vi "Start_track.vi"(0 "TCP connection ID":refnum<k5>, 5 "UDP connection ID":refnum<k16>, 7 "IP address in":u32, 11 "Euler Angles DMARS [º] debug":cluster{"phi":dbl, "theta":dbl, "psi":dbl}={"phi"=2.3, "theta"=1.93, "psi"=0.0}, 12 "error in":errorcluster) -> (4 "TCP connection ID out":refnum<k5>, 6 "UDP connection ID out":refnum<k16>, 8 "IP address out":u32, 10 "timeout ms (25000)":i32=1000, 14 "error out":errorcluster)   [LabVIEW 2017]
panel:
  out "outer ini":string
  out "middle ini":string
  out "inner ini":string
  out "String 5":string
  out "String 4":string
  out "String 3":string
  out "String 2":string
  out "String 1":string
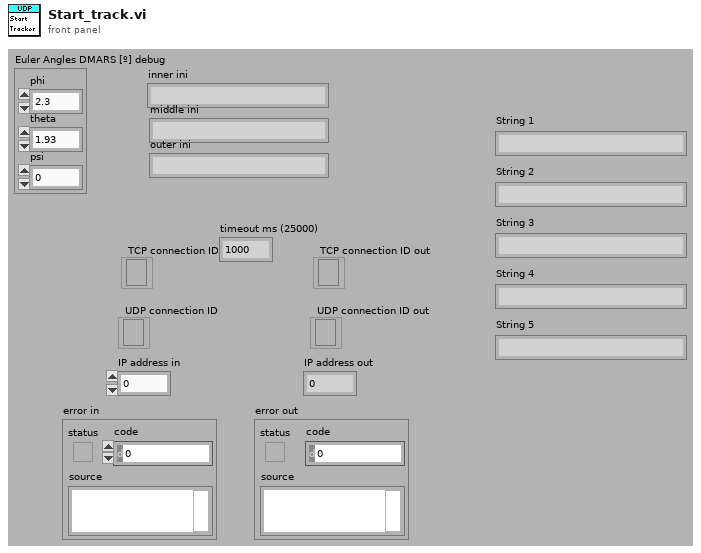
[diagram p1: front panel]
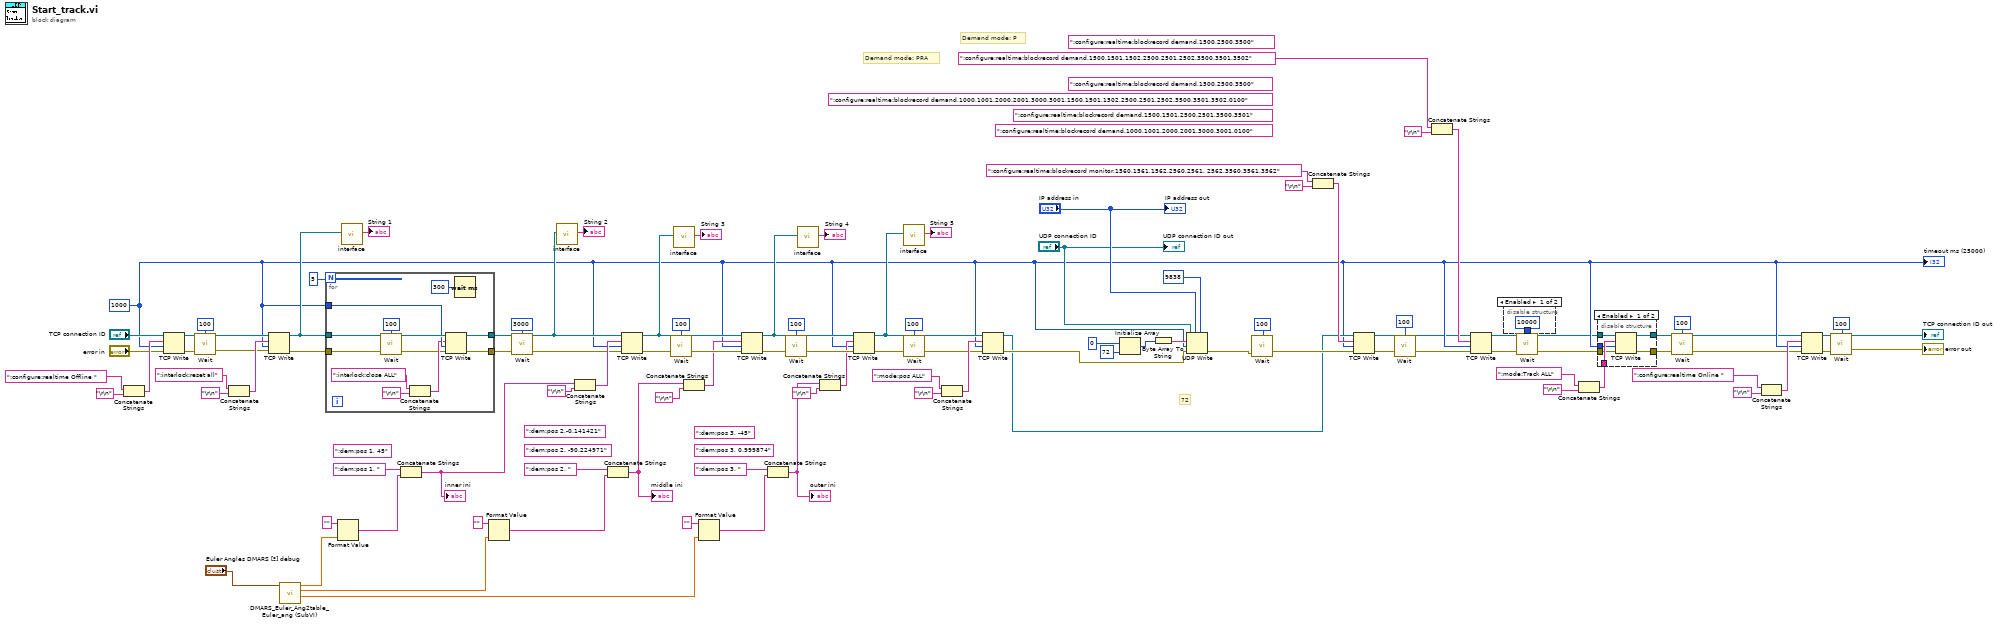
[diagram p0: block diagram]
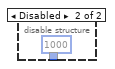
[diagram p3: hidden frame]
diagram:
  (unwired) ":dem:pos 3, 0.999874" ("ACL Command")
  (unwired) ":dem:pos 2, -90.224971" ("ACL Command")
  (unwired) ":dem:pos 3, -45" ("ACL Command")
  (unwired) ":dem:pos 2,-0.141421" ("ACL Command")
  (unwired) ":configure:realtime:blockrecord demand,1500,2500,3500" ("string")
  (unwired) ":configure:realtime:blockrecord demand,1000,1001,2000,2001,3000,3001,1500,1501,1502,2500,2501,2502,3500,3501,3502,0100" ("string")
  (unwired) ":configure:realtime:blockrecord demand,1000,1001,2000,2001,3000,3001,0100" ("string")
  (unwired) ":configure:realtime:blockrecord demand,1500,2500,3500" ("string")
  (unwired) ":configure:realtime:blockrecord demand,1500,1501,2500,2501,3500,3501" ("string")
  (unwired) ":dem:pos 1, 45" ("ACL Command")
  w29 = 1000 ("timeout ms (25000)")
  # "Demand mode: P"
  # "Demand mode: PRA"
  # "72"
  n1 = Concatenate Strings(":configure:realtime Offline " ("ACL Command"), "\r\n") -> (w36:string)
  n2 = TCP Write(connection ID="TCP connection ID", data in=w36, error in (no error)="error in", 9:w29) -> (connection ID out=w33:refnum<k5>, error out=w32:errorcluster)  [unwired: 1 out]
  n3 = call "Wait.vi"("Wartezeit in ms"=u32 100, "error in (no error)"=w32) -> ("error out"=w52:errorcluster)  [unwired: 3 in]
  n4 = Concatenate Strings(":interlock:reset all" ("ACL Command"), "\r\n") -> (w55:string)
  n5 = TCP Write(connection ID=w33, data in=w55, error in (no error)=w52, 9:w29) -> (connection ID out=w75:refnum<k5>, error out=w54:errorcluster)  [unwired: 1 out]
  n6 = call "DMARS_Euler_Ang2table_Euler_ang (SubVI).vi"("Euler Angles DMARS [º] debug"="Euler Angles DMARS [º] debug") -> ("OUTER"=w1:dbl, "MIDDLE"=w2:dbl, "INNER"=w7:dbl)  [unwired: 8 in]
  n7 = for {
    N: 5 -> [_]
    tunnel: w75 -> [w113]
    tunnel: [w112] -> w69
    tunnel: [w111] -> w65
    tunnel: w29 -> [w110]
    tunnel: w54 -> [w106]
    n8 = call "Wait.vi"("Wartezeit in ms"=u32 100, "error in (no error)"=w106) -> ("error out"=w105:errorcluster)  [unwired: 3 in]
    n9 = Concatenate Strings(":interlock:close ALL" ("ACL Command"), "\r\n") -> (w107:string)
    n10 = TCP Write(connection ID=w113, data in=w107, error in (no error)=w105, 9:w110) -> (connection ID out=w112:refnum<k5>, error out=w111:errorcluster)  [unwired: 1 out]
    n11 = Wait (ms)(milliseconds to wait=u32 300) -> ()  [unwired: 1 out]
  }
  n12 = Format Value(string ("")="", value (0)=w7) -> (output string=w14:string)  [unwired: 1 in]
  n13 = call "interface.vi"("TCP Network Connection Refnum"=w75) -> ("String"=→"String 1":string)  [unwired: 8 in, 2 out]
  n14 = Concatenate Strings(":dem:pos 1, " ("ACL Command"), w14) -> (w6:string)
  "inner ini" <- w6
  n15 = Format Value(string ("")="", value (0)=w2) -> (output string=w13:string)  [unwired: 1 in]
  n16 = call "Wait.vi"("Wartezeit in ms"=u32 3000, "error in (no error)"=w65) -> ("error out"=w76:errorcluster)  [unwired: 3 in]
  n17 = call "interface.vi"("TCP Network Connection Refnum"=w69) -> ("String"=→"String 2":string)  [unwired: 8 in, 2 out]
  n18 = Concatenate Strings(w6, "\r\n") -> (w77:string)
  n19 = Concatenate Strings(":dem:pos 2, " ("ACL Command"), w13) -> (w5:string)
  "middle ini" <- w5
  n20 = TCP Write(connection ID=w69, data in=w77, error in (no error)=w76, 9:w29) -> (connection ID out=w68:refnum<k5>, error out=w91:errorcluster)  [unwired: 1 out]
  n21 = call "Wait.vi"("Wartezeit in ms"=u32 100, "error in (no error)"=w91) -> ("error out"=w93:errorcluster)  [unwired: 3 in]
  n22 = call "interface.vi"("TCP Network Connection Refnum"=w68) -> ("String"=→"String 3":string)  [unwired: 8 in, 2 out]
  n23 = Concatenate Strings(w5, "\r\n") -> (w78:string)
  n24 = Format Value(string ("")="", value (0)=w1) -> (output string=w8:string)  [unwired: 1 in]
  n25 = TCP Write(connection ID=w68, data in=w78, error in (no error)=w93, 9:w29) -> (connection ID out=w67:refnum<k5>, error out=w88:errorcluster)  [unwired: 1 out]
  n26 = Concatenate Strings(":dem:pos 3, " ("ACL Command"), w8) -> (w4:string)
  "outer ini" <- w4
  n27 = call "Wait.vi"("Wartezeit in ms"=u32 100, "error in (no error)"=w88) -> ("error out"=w89:errorcluster)  [unwired: 3 in]
  n28 = call "interface.vi"("TCP Network Connection Refnum"=w67) -> ("String"=→"String 4":string)  [unwired: 8 in, 2 out]
  n29 = Concatenate Strings(w4, "\r\n") -> (w79:string)
  n30 = TCP Write(connection ID=w67, data in=w79, error in (no error)=w89, 9:w29) -> (connection ID out=w49:refnum<k5>, error out=w86:errorcluster)  [unwired: 1 out]
  n31 = call "interface.vi"("TCP Network Connection Refnum"=w49) -> ("String"=→"String 5":string)  [unwired: 8 in, 2 out]
  n32 = call "Wait.vi"("Wartezeit in ms"=u32 100, "error in (no error)"=w86) -> ("error out"=w50:errorcluster)  [unwired: 3 in]
  n33 = Concatenate Strings(":mode:pos ALL" ("ACL Command"), "\r\n") -> (w80:string)
  n34 = TCP Write(connection ID=w49, data in=w80, error in (no error)=w50, 9:w29) -> (connection ID out=w46:refnum<k5>, error out=w47:errorcluster)  [unwired: 1 out]
  n35 = Initialize Array(u8 0, 72 ("dimension size")) -> (w97:u8[])
  n36 = Byte Array To String(unsigned byte array=w97) -> (string=w96:string)
  n37 = UDP Write(address="IP address in", port or service name=u16 9838 ("Remote Port"), connection ID="UDP connection ID", data in=w96, 8:w47, 9:w29) -> (error out=w94:errorcluster)  [unwired: 1 out]
  n38 = call "Wait.vi"("Wartezeit in ms"=u32 100, "error in (no error)"=w94) -> ("error out"=w59:errorcluster)  [unwired: 3 in]
  n39 = Concatenate Strings(":configure:realtime:blockrecord monitor,1560,1561,1562,2560,2561, 2562,3560,3561,3562" ("ACL Command"), "\r\n") -> (w64:string)
  n40 = TCP Write(connection ID=w46, data in=w64, error in (no error)=w59, 9:w29) -> (connection ID out=w18:refnum<k5>, error out=w20:errorcluster)  [unwired: 1 out]
  n41 = call "Wait.vi"("Wartezeit in ms"=u32 100, "error in (no error)"=w20) -> ("error out"=w19:errorcluster)  [unwired: 3 in]
  n42 = Concatenate Strings(":configure:realtime:blockrecord demand,1500,1501,1502,2500,2501,2502,3500,3501,3502" ("string"), "\r\n") -> (w61:string)
  n43 = TCP Write(connection ID=w18, data in=w61, error in (no error)=w19, 9:w29) -> (connection ID out=w23:refnum<k5>, error out=w22:errorcluster)  [unwired: 1 out]
  n44 = disable-structure shown="Enabled" {
    disable-tunnel: [u32 10000 ("Wartezeit in ms") u32 1000 ("Wartezeit in ms")] -> w58
    frame Enabled {
    }
    frame Disabled {
    }
  }
  n45 = call "Wait.vi"("Wartezeit in ms"=w58, "error in (no error)"=w22) -> ("error out"=w24:errorcluster)  [unwired: 3 in]
  n46 = Concatenate Strings(":mode:Track ALL" ("ACL Command"), "\r\n") -> (w30:string)
  n47 = disable-structure shown="Enabled" {
    disable-tunnel: w30 -> [w121 _]
    disable-tunnel: w29 -> [w120 _]
    disable-tunnel: [w119 w122] -> w28
    disable-tunnel: [w118 w123] -> w27
    disable-tunnel: w24 -> [w117 w122]
    disable-tunnel: w23 -> [w116 w123]
    frame Enabled {
      n48 = TCP Write(connection ID=w116, data in=w121, error in (no error)=w117, 9:w120) -> (connection ID out=w118:refnum<k5>, error out=w119:errorcluster)  [unwired: 1 out]
    }
    frame Disabled {
    }
  }
  n49 = call "Wait.vi"("Wartezeit in ms"=u32 100, "error in (no error)"=w28) -> ("error out"=w40:errorcluster)  [unwired: 3 in]
  n50 = Concatenate Strings(":configure:realtime Online " ("ACL Command"), "\r\n") -> (w42:string)
  n51 = TCP Write(connection ID=w27, data in=w42, error in (no error)=w40, 9:w29) -> (connection ID out=→"TCP connection ID out":refnum<k5>, error out=w45:errorcluster)  [unwired: 1 out]
  n52 = call "Wait.vi"("Wartezeit in ms"=u32 100, "error in (no error)"=w45) -> ("error out"=→"error out":errorcluster)  [unwired: 3 in]
  "UDP connection ID out" <- "UDP connection ID"
  "IP address out" <- "IP address in"
  "timeout ms (25000)" <- w29
